vi "Transform.vi"(8 "error in (no error)":errorcluster, 11 "XRay CArm in":refnum<class "XRay CArm.lvclass">) -> (0 "error out":errorcluster, 3 "XRay CArm out":refnum<class "XRay CArm.lvclass">)   [LabVIEW 2026, in "XRay CArm.lvclass"]
uses:
  XRay CArm.lvclass
  XRay CArm.lvclass/XRay CArm.ctl
  <vilib>/picture/3D Picture Control/NI_3D Picture Control.lvlib
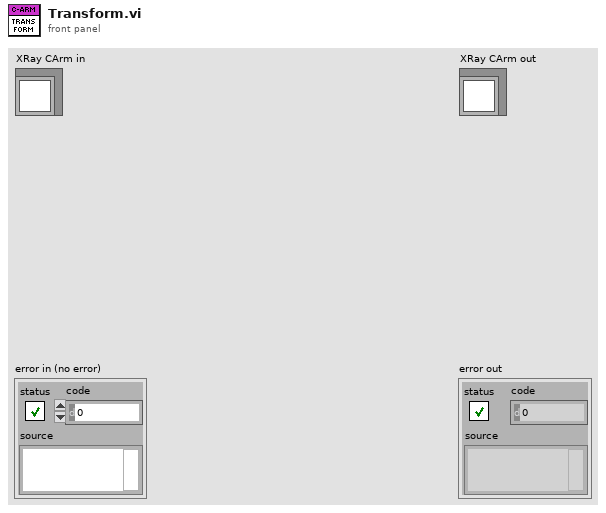
[diagram p1: front panel]
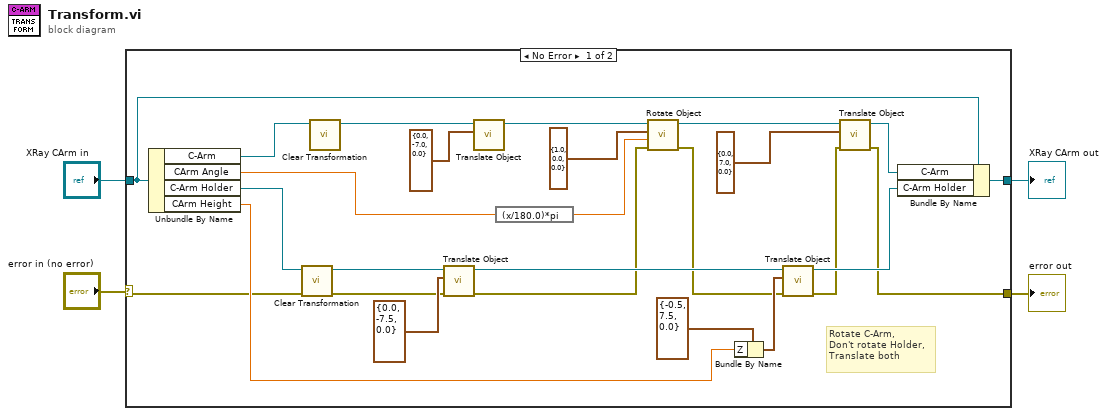
[diagram p0: block diagram]
diagram:
  n1 = case shown="No Error" "error in (no error)" {
    selector: "error in (no error)" -> [w6 w32]
    tunnel: [w7 w32] -> w3
    tunnel: [w29 w31] -> w1
    tunnel: "XRay CArm in" -> [w30 w31]
    frame No Error {
      # "Rotate C-Arm,\nDon't rotate Holder,\nTranslate both"
      n2 = Unbundle By Name(w30) -> ("C-Arm"=w24:refnum<vi>, "CArm Angle"=w10:sgl, "C-Arm Holder"=w23:refnum<vi>, "CArm Height"=w8:sgl)
      n3 = call <vilib>:"Clear Transformation.vi"("error in (no error)"=w6, "Object Refnum In"=w23) -> ("error out"=w5:errorcluster, "Object Refnum Out"=w26:refnum<vi>)  [unwired: 8 out]
      n4 = call <vilib>:"Clear Transformation.vi"("Object Refnum In"=w24) -> ("Object Refnum Out"=w16:refnum<vi>)  [unwired: 1 in, 9 out]
      n5 = call <vilib>:"Translate Object.vi"("error in (no error)"=w5, "Translation"=cluster{"X":sgl, "Y":sgl, "Z":sgl} {"X"=0.0, "Y"=-7.5, "Z"=0.0} ("Translation 4"), "Scene.Object In"=w26) -> ("error out"=w14:errorcluster, "Scene.Object Out"=w21:refnum<vi>)  [unwired: 7 in]
      n6 = call <vilib>:"Translate Object.vi"("Translation"=cluster{"X":sgl, "Y":sgl, "Z":sgl} {"X"=0.0, "Y"=-7.0, "Z"=0.0} ("Translation 3"), "Scene.Object In"=w16) -> ("Scene.Object Out"=w15:refnum<vi>)  [unwired: 8 in, 1 out]
      n7 = expression code="(x/180.0)*pi" ("degrees to radians")(w10) -> (w9:sgl)
      n8 = call <vilib>:"Rotate Object.vi"("error in (no error)"=w14, "Angle"=w9, "Axis"=cluster{"X":sgl, "Y":sgl, "Z":sgl} {"X"=1.0, "Y"=0.0, "Z"=0.0}, "Scene.Object In"=w15) -> ("error out"=w13:errorcluster, "Scene.Object Out"=w20:refnum<vi>)  [unwired: 6 in]
      n9 = Bundle By Name(cluster=cluster{"X":sgl, "Y":sgl, "Z":sgl} {"X"=-0.5, "Y"=7.5, "Z"=0.0} ("Translation"), "Z"=w8) -> (w27:cluster{"X":sgl, "Y":sgl, "Z":sgl})
      n10 = call <vilib>:"Translate Object.vi"("error in (no error)"=w13, "Translation"=w27, "Scene.Object In"=w21) -> ("error out"=w12:errorcluster, "Scene.Object Out"=w22:refnum<vi>)  [unwired: 7 in]
      n11 = call <vilib>:"Translate Object.vi"("error in (no error)"=w12, "Translation"=cluster{"X":sgl, "Y":sgl, "Z":sgl} {"X"=0.0, "Y"=7.0, "Z"=0.0} ("Translation 2"), "Scene.Object In"=w20) -> ("error out"=w7:errorcluster, "Scene.Object Out"=w19:refnum<vi>)  [unwired: 7 in]
      n12 = Bundle By Name(cluster=w30, "C-Arm"=w19, "C-Arm Holder"=w22) -> (w29:refnum<class "XRay CArm.lvclass">)
    }
    frame Error {
    }
  }
  "error out" <- w3
  "XRay CArm out" <- w1
